vi "Listbox Select.vi"(8 "error in (no error)":errorcluster, 11 "Loop data in":T1={"Config"={"List"=[], "max rows"=8, "Listbox placement"=enum."None", "String Color Options"={"Use? (F)"=FALSE, "Color - Valid"=0, "Color - Invalid"=0, "Allow blank?"=FALSE}}, "Refs"={"String"=refnum, "Listbox"=refnum}, "State"={"LB active?"=FALSE}}) -> (0 "error out":errorcluster, 3 "Loop data out":T1={"Config"={"List"=[], "max rows"=8, "Listbox placement"=enum."None", "String Color Options"={"Use? (F)"=FALSE, "Color - Valid"=0, "Color - Invalid"=0, "Allow blank?"=FALSE}}, "Refs"={"String"=refnum, "Listbox"=refnum}, "State"={"LB active?"=FALSE}})   [LabVIEW 2021, in "Autocomplete Textbox.lvlib"]
uses:
  Autocomplete Textbox.lvlib
  Loop Data.ctl
  Inputs.ctl
  Classes/Handle/Listbox placement.ctl
  Color String Options.ctl
  Refs.ctl
  State data.ctl
  Classes/Handle/Handle.lvclass
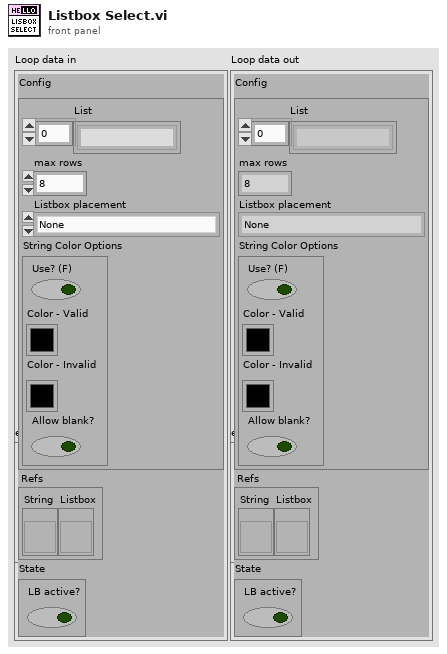
[diagram p1: front panel]
types:
  T1 = typedef "Autocomplete Textbox.lvlib/Loop Data.ctl" = cluster{"Config":T2, "Refs":T5, "State":T6}
  T2 = typedef "Autocomplete Textbox.lvlib/Inputs.ctl" = cluster{"List":string[], "max rows":i32, "Listbox placement":T3, "String Color Options":T4}
  T3 = typedef "Autocomplete Textbox.lvlib/Handle.lvclass/Listbox placement.ctl" = enum16{"None", "Under String", "Fit to Pane"}
  T4 = typedef "Autocomplete Textbox.lvlib/Color String Options.ctl" = cluster{"Use? (F)":bool, "Color - Valid":u32, "Color - Invalid":u32, "Allow blank?":bool}
  T5 = typedef "Autocomplete Textbox.lvlib/Refs.ctl" = cluster{"String":refnum<vi>, "Listbox":refnum<vi>}
  T6 = typedef "Autocomplete Textbox.lvlib/State data.ctl" = cluster{"LB active?":bool}
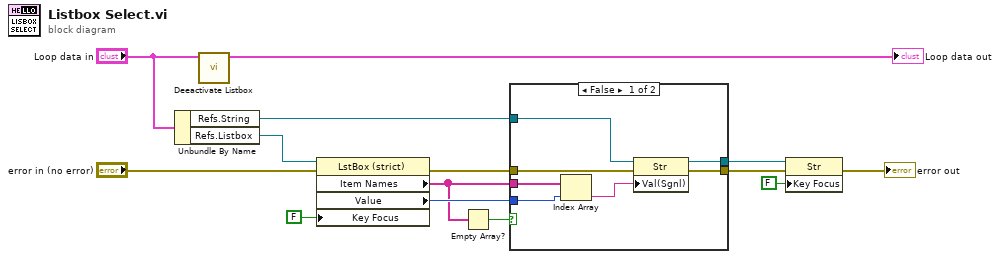
[diagram p0: block diagram]
diagram:
  n1 = Unbundle By Name("Loop data in") -> ("Refs.String"=w9:refnum<vi>, "Refs.Listbox"=w12:refnum<vi>)
  n2 = call "Deeactivate Listbox.vi"("Loop data in"="Loop data in") -> ("Loop data out"=→"Loop data out":T1)  [unwired: 9 in, 1 out]
  n3 = property class="LstBox (strict)"(reference=w12, error in="error in (no error)", "Key Focus"=FALSE ("Visible")) -> (error out=w11:errorcluster, "Item Names"=w2:string[], "Value"=w13:i32)  [unwired: 1 out]
  n4 = Empty Array?(array=w2) -> (empty?=w1:bool)
  n5 = case shown="False" w1 {
    tunnel: w13 -> [w21 _]
    tunnel: w11 -> [w19 w23]
    tunnel: w9 -> [w18 w22]
    tunnel: [w17 w23] -> w6
    tunnel: [w16 w22] -> w5
    tunnel: w2 -> [w15 _]
    frame False {
      n6 = Index Array(array=w15, index=w21) -> (element=w20:string)
      n7 = property class="Str"(reference=w18, error in=w19, "Val(Sgnl)"=w20) -> (reference out=w16:refnum<vi>, error out=w17:errorcluster)
    }
    frame True {
    }
  }
  n8 = property class="Str"(reference=w5, error in=w6, "Key Focus"=FALSE) -> (error out=→"error out":errorcluster)  [unwired: 1 out]
